vi "MutationOptionsErrorCheck.vi"(8 "error in (no error)":errorcluster, 10 "Mutation Options":T1, 11 "Mutation Record":T2 {"LabVIEW Version" format="%.0x"}) -> (0 "error out":errorcluster, 3 "Mutation Record":T2 {"LabVIEW Version" format="%.0x"})   [LabVIEW 2019, in "BlueSerialization.lvlib" / "BlueSerializer.lvclass"]
uses:
  BlueSerializer.lvclass
  <vilib>/Utility/EditLVLibs/LVClass/Mutation Record.ctl
  <vilib>/Utility/EditLVLibs/LibVersion.ctl
  DeserializeMutationOptions.ctl
  <vilib>/Utility/error.llb/Error Cluster From Error Code.vi
  <vilib>/ErrorRing/Error Ring.xnode
  <vilib>/Utility/EditLVLibs/Edit LVLibs.lvlib
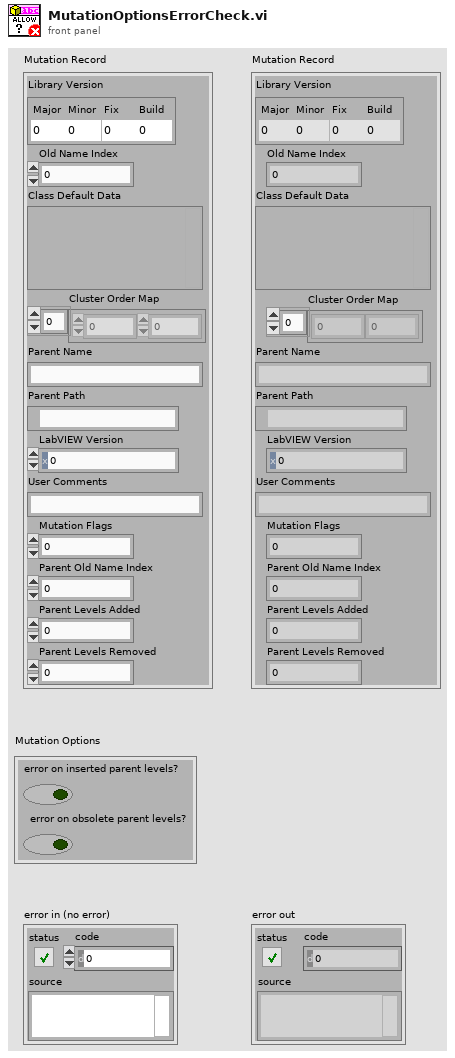
[diagram p1: front panel]
types:
  T1 = typedef "BlueSerialization.lvlib/BlueSerializer.lvclass/DeserializeMutationOptions.ctl" = cluster{"error on inserted parent levels?":bool, "\terror on obsolete parent levels?":bool}
  T2 = typedef "Edit LVLibs.lvlib/Mutation Record.ctl" = cluster{"Library Version":T3, "Old Name Index":u8, "Class Default Data":variant, "Cluster Order Map":u32[], "Parent Name":string, "Parent Path":path, "LabVIEW Version":u32, "User Comments":string, "Mutation Flags":u8, "Parent Old Name Index":u8, "Parent Levels Added":u16, "Parent Levels Removed":u16}
  T3 = typedef "Edit LVLibs.lvlib/LibVersion.ctl" = cluster{"Major":u16, "Minor":u16, "Fix":u16, "Build":u16}
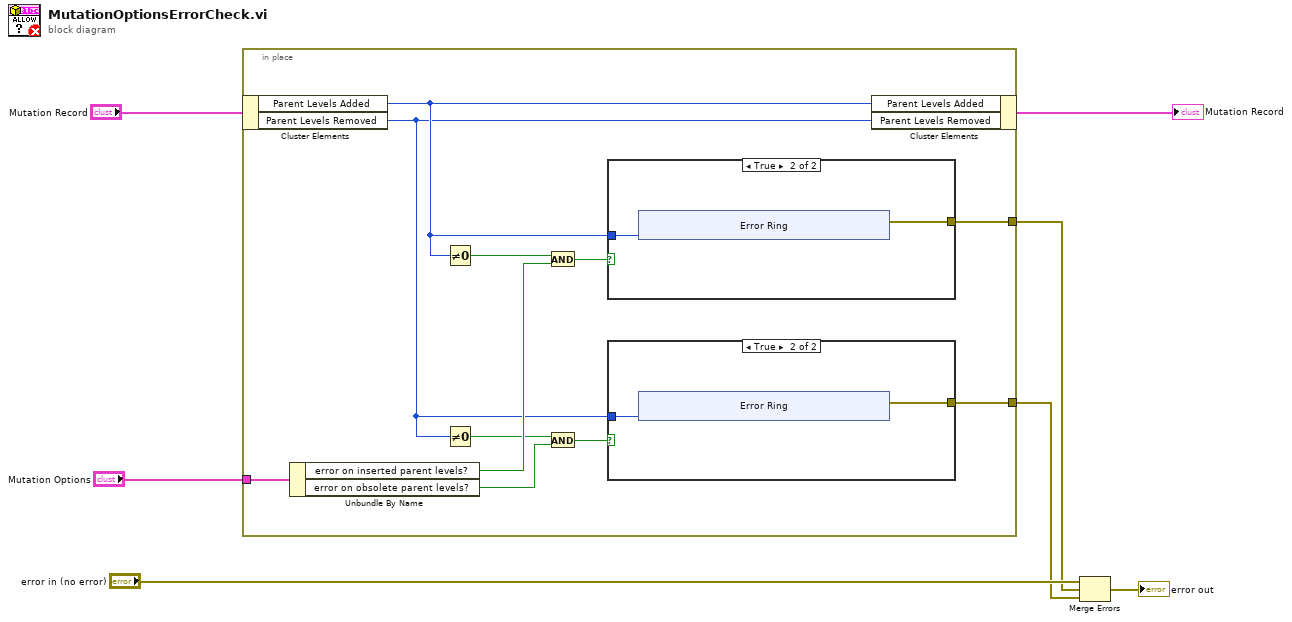
[diagram p0: block diagram]
diagram:
  n1 = in-place {
    in-place-border: "Mutation Options" -> [w18]
    in-place-border: [w9] -> w3
    in-place-border: [w8] -> w2
    n2 = in-place-cluster #1("Mutation Record") -> ("Parent Levels Added"=w14:u16, "Parent Levels Removed"=w10:u16)
    n3 = Unbundle By Name(w18) -> ("error on inserted parent levels?"=w17:bool, "error on obsolete parent levels?"=w11:bool)
    n4 = Not Equal To 0?(x=w14) -> (x != 0?=w16:bool)
    n5 = Not Equal To 0?(x=w10) -> (x != 0?=w12:bool)
    n6 = And(x=w16, y=w17) -> (x .and. y?=w15:bool)
    n7 = And(x=w12, y=w11) -> (x .and. y?=w13:bool)
    n8 = case shown="True" w15 {
      tunnel: w14 -> [_ w29]
      tunnel: [_ w28] -> w9
      frame False {
      }
      frame True {
        n9 = xnode "Error Ring"("parameter 0"=w29) -> ("error out"=w28:errorcluster)
      }
    }
    n10 = case shown="True" w13 {
      tunnel: w10 -> [_ w20]
      tunnel: [_ w19] -> w8
      frame False {
      }
      frame True {
        n11 = xnode "Error Ring"("parameter 0"=w20) -> ("error out"=w19:errorcluster)
      }
    }
    n12 = in-place-cluster #1("Parent Levels Added"=w14, "Parent Levels Removed"=w10) -> (→"Mutation Record":T2)
  }
  n13 = Merge Errors("error in (no error)", w3, w2) -> (→"error out":errorcluster)
